vi "Open Connection.vi"(8 "error in (no error)":errorcluster, 10 "Connection Info (Member Data/Prompt)":variant, 11 "ODBC in":refnum<class "ADODB.lvclass">) -> (0 "error out":errorcluster, 3 "ODBC out":refnum<class "ADODB.lvclass">)   [LabVIEW 2020, in "ADODB.lvlib" / "ADODB.lvclass"]
uses:
  ADODB.lvclass
  ADODB.lvclass/ADODB.ctl
  Read Connection Information.vi
  <vilib>/addons/database/Connection.llb/DB Tools Open Connec (Path).vi
  <vilib>/Utility/Data Type/NI_Data Type.lvlib
  <vilib>/addons/database/NI_Database_API.lvlib
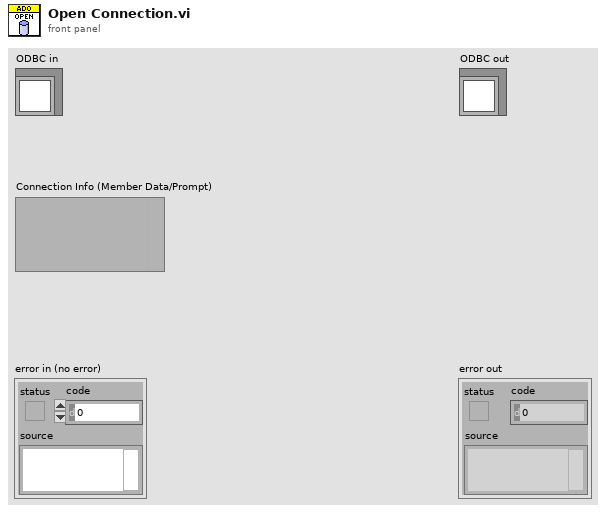
[diagram p1: front panel]
types:
  T1 = typedef "NI_Data Type.lvlib/Data Type.ctl" = enum8{"Invalid Type", "Void", "I8", "I16", "I32", "I64", "U8", "U16", "U32", "U64", "Single Float", "Double Float", "Extended Float", "Single Complex", "Double Complex", "Extended Complex", "Enum U8", "Enum U16", "Enum U32", "Enum U64", "Single Float With Unit", "Double Float With Unit", "Extended Float With Unit", "Single Complex with Unit", "Double Complex with Unit", "Extended Complex with Unit", "Boolean", "String", "Path", "Picture", "Tag", "Array", "Cluster", "Variant", "LV Variant", "Waveform", "Timestamp", "Digital Waveform", "Digital Data", "ExpressData", "Refnum", "External Data", "VI", "Poly VI", "LabVIEW Class Instance", "Fixed Point", "Set Collection", "Map Collection"}
  T2 = typedef "NI_Database_API.lvlib/Conn ObjectReference.ctl" = refnum<k1>
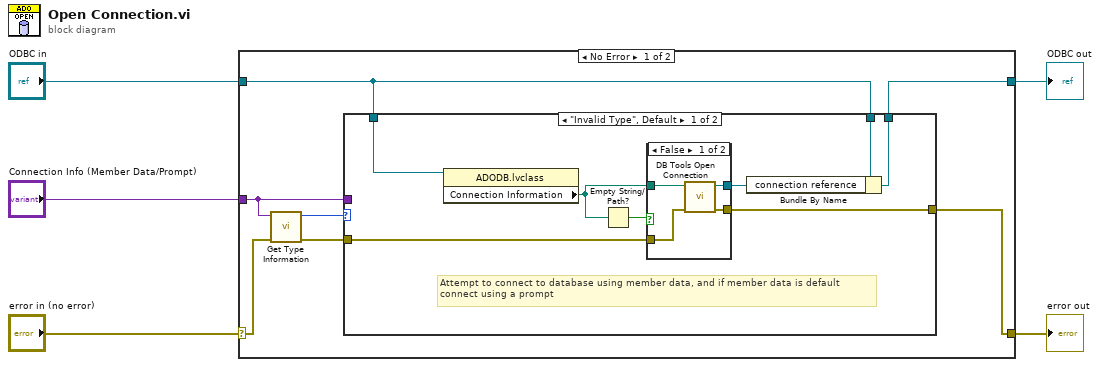
[diagram p0: block diagram]
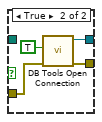
[diagram p2: hidden frame]
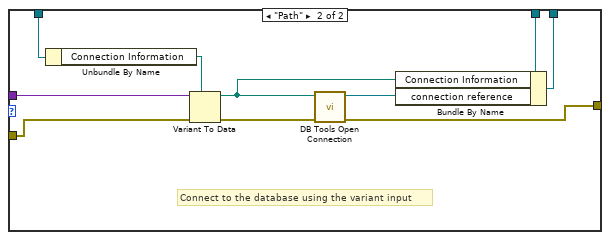
[diagram p3: hidden frame]
diagram:
  n1 = case shown="No Error" "error in (no error)" {
    selector: "error in (no error)" -> [w8 w40]
    tunnel: [w6 w40] -> w4
    tunnel: "ODBC in" -> [w10 w39]
    tunnel: [w9 w39] -> w2
    tunnel: "Connection Info (Member Data/Prompt)" -> [w11 _]
    frame No Error {
      n2 = call <vilib>:"Get Type Information.vi"("error in (no error)"=w8, "variant"=w11) -> ("error out"=w7:errorcluster, "type"=w12:T1)  [unwired: 5 in, 3 out]
      n3 = case shown="\"Invalid Type\", Default" w12 {
        tunnel: w11 -> [_ w37]
        tunnel: w10 -> [w14 w38]
        tunnel: w10 -> [w20 w34]
        tunnel: [w19 w33] -> w9
        tunnel: w7 -> [w17 w35]
        tunnel: [w16 w31] -> w6
        frame "Invalid Type", Default {
          # "Attempt to connect to database using member data, and if member data is default\nconnect using a prompt"
          n4 = property class="ADODB.lvclass"(reference=w14) -> ("Connection Information"=w13:path)  [unwired: 1 in, 2 out]
          n5 = Empty String/Path?(string/path=w13) -> (empty?=w18:bool)
          n6 = case shown="False" w18 {
            tunnel: [w24 w28] -> w15
            tunnel: w17 -> [w23 w26]
            tunnel: [w22 w25] -> w16
            tunnel: w13 -> [w21 _]
            frame False {
              n7 = call-poly <vilib>:"DB Tools Open Connection.vi"("error in (no error)"=w23, "connection information"=w21) -> ("error out"=w22:errorcluster, "connection reference"=w24:T2)  [unwired: 6 in]
            }
            frame True {
              n8 = call-poly <vilib>:"DB Tools Open Connection.vi"("error in (no error)"=w26, "prompt? (F)"=TRUE) -> ("error out"=w25:errorcluster, "connection reference"=w28:T2)  [unwired: 6 in]
            }
          }
          n9 = Bundle By Name(cluster=w20, "connection reference"=w15) -> (w19:refnum<class "ADODB.lvclass">)
        }
        frame "Path" {
          # "Connect to the database using the variant input"
          n10 = Unbundle By Name(w38) -> ("Connection Information"=w36:path)
          n11 = Variant To Data(error in=w35, type=w36, Variant=w37) -> (data=w29:path, error out=w32:errorcluster)
          n12 = call-poly <vilib>:"DB Tools Open Connection.vi"("error in (no error)"=w32, "connection information"=w29) -> ("error out"=w31:errorcluster, "connection reference"=w30:T2)  [unwired: 6 in]
          n13 = Bundle By Name(cluster=w34, "Connection Information"=w29, "connection reference"=w30) -> (w33:refnum<class "ADODB.lvclass">)
        }
      }
    }
    frame Error {
    }
  }
  "error out" <- w4
  "ODBC out" <- w2
